vi "Field Draw Targets.vi"(4 "Lado":enum16{"Esquerdo", "Direito"}(ring) caption="Enum", 6 "Draw Targets?":T1, 8 "Picture In":picture, 9 "Offset":cluster{"Width":dbl, "Height":dbl}, 10 "Scale":dbl, 11 "our_robots":T2[](array[typedef])) -> (0 "Picture Out":picture, 1 "Offset Out":cluster{"Width":dbl, "Height":dbl}, 2 "Scale Out":dbl)   [LabVIEW 2018]
uses:
  Controls/AI Robot.ctl
  Controls/Functions Enum.ctl
  Controls/AttackerStates.ctl
  Controls/PathDests.ctl
  Controls/PathDest.ctl
  git/SSLView/DrawTargets.ctl
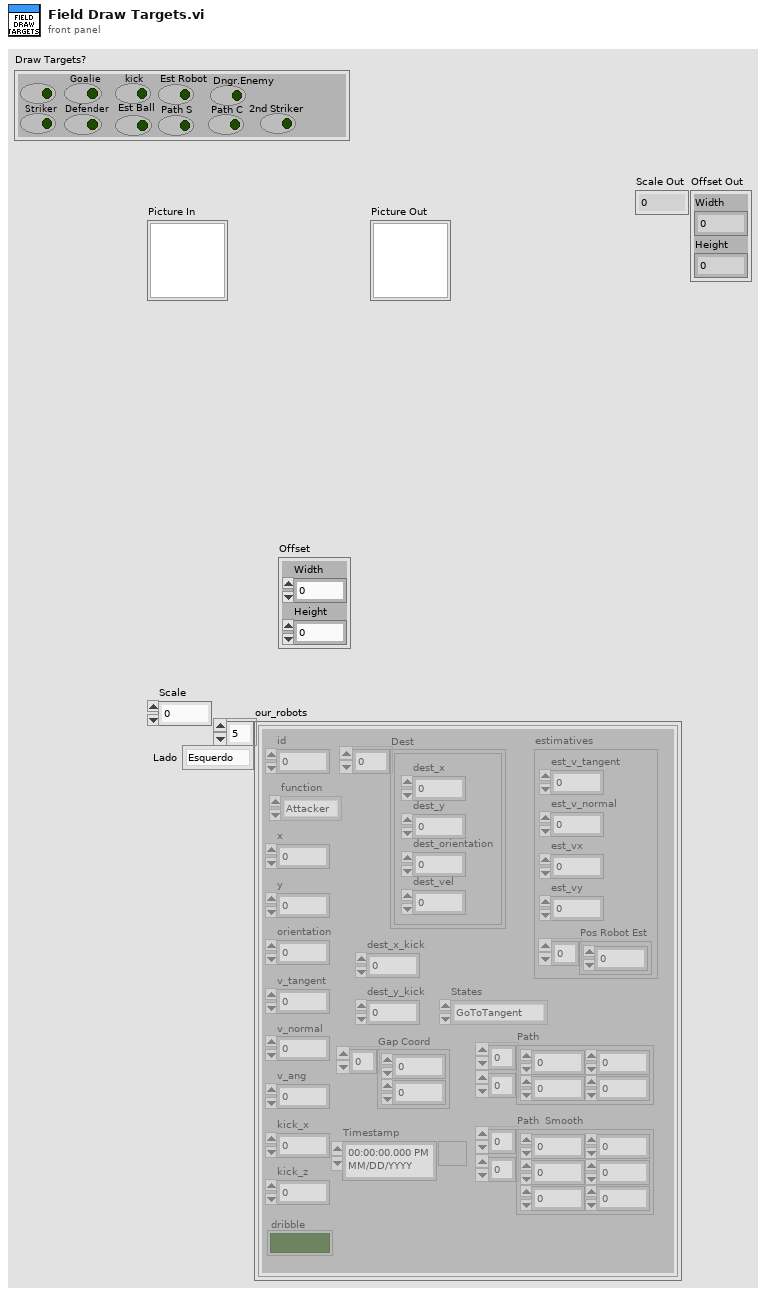
[diagram p1: front panel]
types:
  T1 = typedef "DrawTargets.ctl" = cluster{"Attacker":bool, "Striker":bool, "Goalie":bool, "Defender":bool, "kick":bool, "Est Ball":bool, "Est Robot":bool, "Path S":bool, "Path C":bool, "Dngr.Enemy":bool, "2nd Striker":bool}
  T2 = typedef "AI Robot.ctl" = cluster{"id":u32, "function":T3, "x":dbl, "y":dbl, "orientation":dbl, "v_tangent":dbl, "v_normal":dbl, "v_ang":dbl, "kick_x":dbl, "kick_z":dbl, "dribble":bool, "Timestamp":timestamp, "estimatives":cluster{"est_v_tangent":dbl, "est_v_normal":dbl, "est_vx":dbl, "est_vy":dbl, "Pos Robot Est":dbl[]}, "dest_x_kick":dbl, "dest_y_kick":dbl, "Gap Coord":dbl[], "States":T4, "Path ":dbl[][], "Path  Smooth":dbl[][], "Dest":T5}
  T3 = typedef "Functions Enum.ctl" = enum16{"2nd Striker", "Attacker", "Goalie", "Defender", "Striker", "Goto 0", "Dummy", "Kicker", "ZigZag 0", "ZigZag 1", "ZigZag 2", "ZigZag 3", "ZigZag 4", "ZigZag 5", "ZigZag 6", "ZigZag 7", "ZigZag 8", ""}
  T4 = typedef "AttackerStates.ctl" = enum16{"Pass", "GoToTangent", "BallGetting", "GoToKick", ""}
  T5 = typedef "PathDests.ctl" = T6[]
  T6 = typedef "PathDest.ctl" = cluster{"dest_x":dbl, "dest_y":dbl, "dest_orientation":dbl, "dest_vel":dbl}
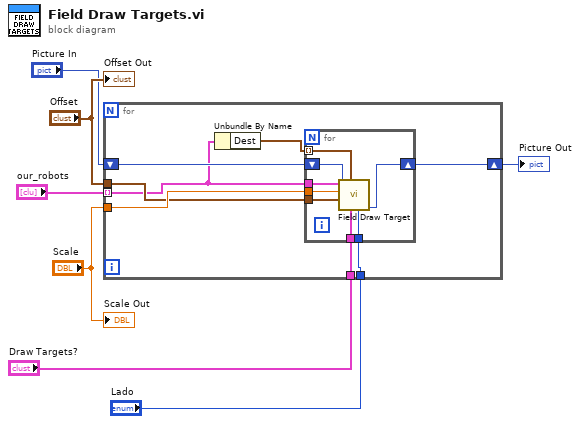
[diagram p0: block diagram]
diagram:
  n1 = for {
    tunnel: "Scale" -> [w15]
    tunnel: "Offset" -> [w13]
    shift-right: [w14] -> w4
    shift-left: "Picture In" -> [w12]
    tunnel: "our_robots" -> [w9] mode=indexing
    tunnel: "Draw Targets?" -> [w11]
    tunnel: "Lado" -> [w10]
    n2 = Unbundle By Name(w9) -> ("Dest"=w8:T5)
    n3 = for {
      tunnel: w15 -> [w23]
      tunnel: w13 -> [w21]
      tunnel: w9 -> [w19]
      tunnel: w11 -> [w18]
      tunnel: w10 -> [w17]
      shift-right: [w22] -> w14
      shift-left: w12 -> [w20]
      tunnel: w8 -> [w16] mode=indexing
      n4 = call "Field Draw Target.vi"("Lado"=w17, "Draw Targets?"=w18, "Dest"=w16, "picture in"=w20, "Offset"=w21, "Scale mm/pixel"=w23, "Robot"=w19) -> ("picture out"=w22:picture)  [unwired: 4 in]
    }
  }
  "Picture Out" <- w4
  "Scale Out" <- "Scale"
  "Offset Out" <- "Offset"
